vi "svfa_Compute FFT Spectrum.vi"(2 "sampling frequency [Hz]":dbl=10000.0 format="%.2f", 3 "signal [EU]":dbl[](array[numeric]) format="%.2f") -> (0 "df [Hz]":dbl format="%.2f", 1 "FFT spectrum [EUrms]":cdb[](array[numeric]) format="%.2f")   [LabVIEW 2017]
uses:
  <vilib>/Analysis/2dsp.llb/Real FFT.vi
  <vilib>/Analysis/NI_AALPro.lvlib
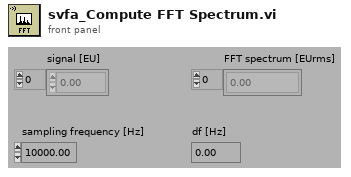
[diagram p1: front panel]
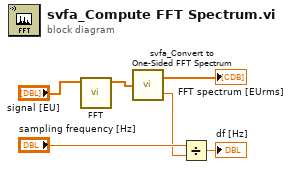
[diagram p0: block diagram]
diagram:
  n1 = call-poly <vilib>:"FFT.vi"("X"="signal [EU]") -> ("FFT {X}"=w3:cdb[])  [unwired: 9 in, 1 out]
  n2 = call <vilib>:"svfa_Convert to One-Sided FFT Spectrum.vi"("two-sided FFT spectrum"=w3) -> ("one-sided FFT spectrum"=→"FFT spectrum [EUrms]":cdb[], "block size"=w1:dbl)
  n3 = Divide(x="sampling frequency [Hz]", y=w1) -> (x/y=→"df [Hz]":dbl)
